vi "2019-05-013_SequenceStructure_01.vi"() -> ()   [LabVIEW 2018]
panel:
  out "Which Button?":T1(ring)
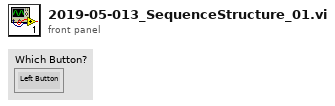
[diagram p1: front panel]
types:
  T1 = enum16{"Left Button", "Center Button", "Right Button", "Window Close"}
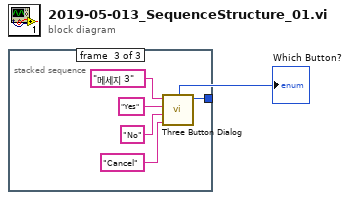
[diagram p0: block diagram]
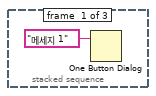
[diagram p2: hidden frame]
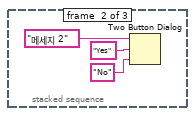
[diagram p3: hidden frame]
diagram:
  n1 = stacked-sequence {
    tunnel: [_ _ w6] -> w1
    frame #0 {
      n2 = One Button Dialog(message="메세지 1" ("메시지")) -> ()  [unwired: 1 in, 1 out]
    }
    frame #1 {
      n3 = Two Button Dialog(message="메세지 2" ("메시지"), 1:"No" ("거짓 버튼 이름(\"취소\")"), 2:"Yes" ("참 버튼 이름(\"확인\")")) -> ()  [unwired: 1 out]
    }
    frame #2 {
      n4 = call <vilib>:"Three Button Dialog.vi"("Right Button Text (\"Cancel\")"="Cancel" ("Right Button Text (\"Cancel\")"), "Center Button Text (\"No\")"="No" ("Center Button Text (\"No\")"), "Left Button Text (\"Yes\")"="Yes" ("Left Button Text (\"Yes\")"), "message"="메세지 3" ("메시지")) -> ("Which Button?"=w6:T1)  [unwired: 7 in]
    }
  }
  "Which Button?" <- w1
